vi "GetDataPackage_CAN.vi"(8 "error in (no error)":errorcluster, 11 "VISA Refnum in":refnum<visa-resource-name>) -> (0 "error out":errorcluster, 1 "Raw Data":string, 2 "Data":T1[](array[typedef]), 3 "VISA Refnum out":refnum<visa-resource-name>)   [LabVIEW 2020, in "OXYGEN_Datastream.lvlib"]
uses:
  OXYGEN_Datastream.lvlib
  TypeDefs/DataPoint_CAN.ctl
  TypeDefs/CAN_Data.ctl
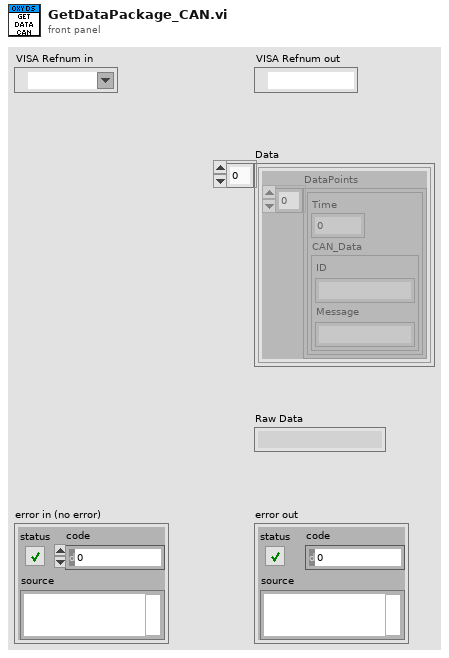
[diagram p1: front panel]
types:
  T1 = typedef "OXYGEN_Datastream.lvlib/DataPoint_CAN.ctl" = cluster{"DataPoints":cluster{"Time":dbl, "CAN_Data":T2}[]}
  T2 = typedef "OXYGEN_Datastream.lvlib/CAN_Data.ctl" = cluster{"ID":string, "Message":string}
  T3 = typedef "OXYGEN_Datastream.lvlib/DataPoint_Variant.ctl" = cluster{"DataPoints":cluster{"Time":dbl, "Value":variant}[]}
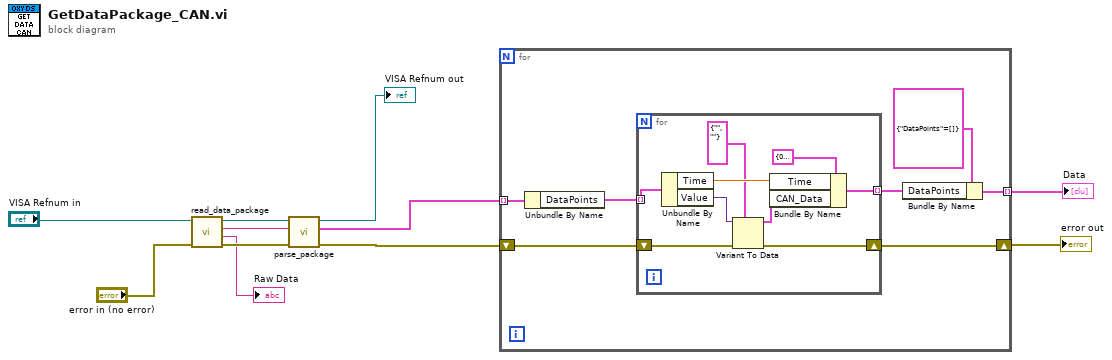
[diagram p0: block diagram]
diagram:
  n1 = call "read_data_package.vi"("error in (no error)"="error in (no error)", "OXY_SCPI Reseource In"="VISA Refnum in") -> ("error out"=w6:errorcluster, "Complete Raw data"=→"Raw Data":string, "Package without Header"=w8:string, "OXY_SCPI Reseource Out"=w7:refnum<visa-resource-name>)  [unwired: 6 in]
  n2 = call "parse_package.vi"("error in (no error)"=w6, "Raw Package without Header"=w8, "OXY_SCPI Reseource In"=w7) -> ("error out"=w4:errorcluster, "DataAllChannels"=w5:T3[], "OXY_SCPI Reseource Out"=→"VISA Refnum out":refnum<visa-resource-name>)  [unwired: 6 in]
  n3 = for {
    tunnel: w5 -> [w18] mode=indexing
    shift-right: [w15] -> w3
    shift-left: w4 -> [w16]
    tunnel: [w14] -> w2 mode=indexing
    n4 = Unbundle By Name(w18) -> ("DataPoints"=w17:cluster{"Time":dbl, "Value":variant}[])
    n5 = for {
      tunnel: w17 -> [w27] mode=indexing
      shift-right: [w24] -> w15
      shift-left: w16 -> [w25]
      tunnel: [w23] -> w13 mode=indexing
      n6 = Unbundle By Name(w27) -> ("Time"=w26:dbl, "Value"=w22:variant)
      n7 = Variant To Data(error in=w25, type=T2 {"ID"="", "Message"=""} ("CAN_Data"), Variant=w22) -> (data=w21:T2, error out=w24:errorcluster)
      n8 = Bundle By Name(cluster=cluster{"Time":dbl, "CAN_Data":T2} {"Time"=0.0, "CAN_Data"={"ID"="", "Message"=""}}, "Time"=w26, "CAN_Data"=w21) -> (w23:cluster{"Time":dbl, "CAN_Data":T2})
    }
    n9 = Bundle By Name(cluster=T1 {"DataPoints"=[]} ("Data"), "DataPoints"=w13) -> (w14:T1)
  }
  "error out" <- w3
  "Data" <- w2
